vi "HoloPy_Example.vi"() -> ()   [LabVIEW 2023, in "holoPyTracks.lvlib"]
uses:
  holoPyTracks.lvlib
  subVis/HologramInfo.ctl
  subVis/analyse_parameters.ctl
panel:
  out "return value 2":sgl[][](array[numeric])
  out "2D Picture 3":picture
  out "2D Picture 2":picture
  out "return value":string
  out "data volume":cluster{"mean":dbl, "std var":dbl}
  out "2D Picture":picture
  in  "directory path":path=path "C:/TRAVAIL/developpement/imagesHolo/20um_bon_40X"
  in  "analyse parameters":T1={"propagation"={"distance ini"=0.0, "number of planes"=100, "step"=1e-06}, "Focus"={"Type"=enum."TENENGRAD", "Sum size"=20}, "Binarisation"={"Threshold ( N x Standard deviation)"=10.0, "Computed on"=enum."1st hologram"}, "CCL"={"Connectivity"=enum."6", "min voxel"=1.0, "max voxel"=1.0}, "Fourier BP filter (pix)"={"High pass (0=none)"=15.0, "Low Pass (0=none)"=125.0}} {"Fourier BP filter (pix)"."Low Pass (0=none)" format="%#_6e"; "CCL"."max voxel" min=1.0 max=100.0; "CCL"."min voxel" min=1.0 max=100.0; "Binarisation"."Threshold ( N x Standard deviation)" min=1.0 max=100.0; "Focus"."Sum size" min=1 max=100; "propagation"."step" format="%#_6e"; "propagation"."distance ini" format="%#_6e"}
  in  "Holo parameters":T2={"wavelength"=6.6e-07, "optical index"=1.33, "Holo size X"=1024, "Holo size Y"=1024, "pixel size"=7e-06, "objective magnification"=40.0} {"wavelength" format="%#_6e"}
  in  "image path":path=path "C:/TRAVAIL/developpement/imagesHolo/20um_bon_40X/20um_40x_int_.7ajp1c6t.000000.bmp"
  in  "error in (no error)":errorcluster
  in  "Python version":string="3.10"
  out "error out":errorcluster
  # "Python Node in holoPY.lvlib:HoloPy_Find_Features.vi->holoPY.lvlib:HoloPy_Example.vi<APPEND>\n\nModule Path: C:\\TRAVAIL\\developpement\\Holo_Python\\Holo_Python_Labview_wrapper.py\nFunction Name: LV_find_features\nPython returned the following error: <class 'ValueError'>\nOnly 6, 18, and 26 connectivities are supported for 3D images. Got: 0\n\n\nCall Stack information:\n  File \"C:\\TRAVAIL\\developpement\\Holo_Python\\Holo_Python_Labview_wrapper.py\", line 294, in LV_find_features\n    h_labels, number_of_labels, statsCCL3D = CCL3D(d_bin_volume_focus, d_volume_module, type_threshold.THRESHOLD, threshold, n_connectivity)\n  File \"C:\\TRAVAIL\\developpement\\Holo_Python\\CCL3D.py\", line 166, in CCL3D\n    labels, number_of_labels = cc3d.connected_components(h_bin_volum, connectivity=n_connectivity, out_dtype=np.uint16, return_N=True)\n  File \"cc3d.pyx\", line 273, in cc3d.connected_components\n\nValueError: Only 6, 18, and 26 connectivities are supported for 3D images. Got: 0"
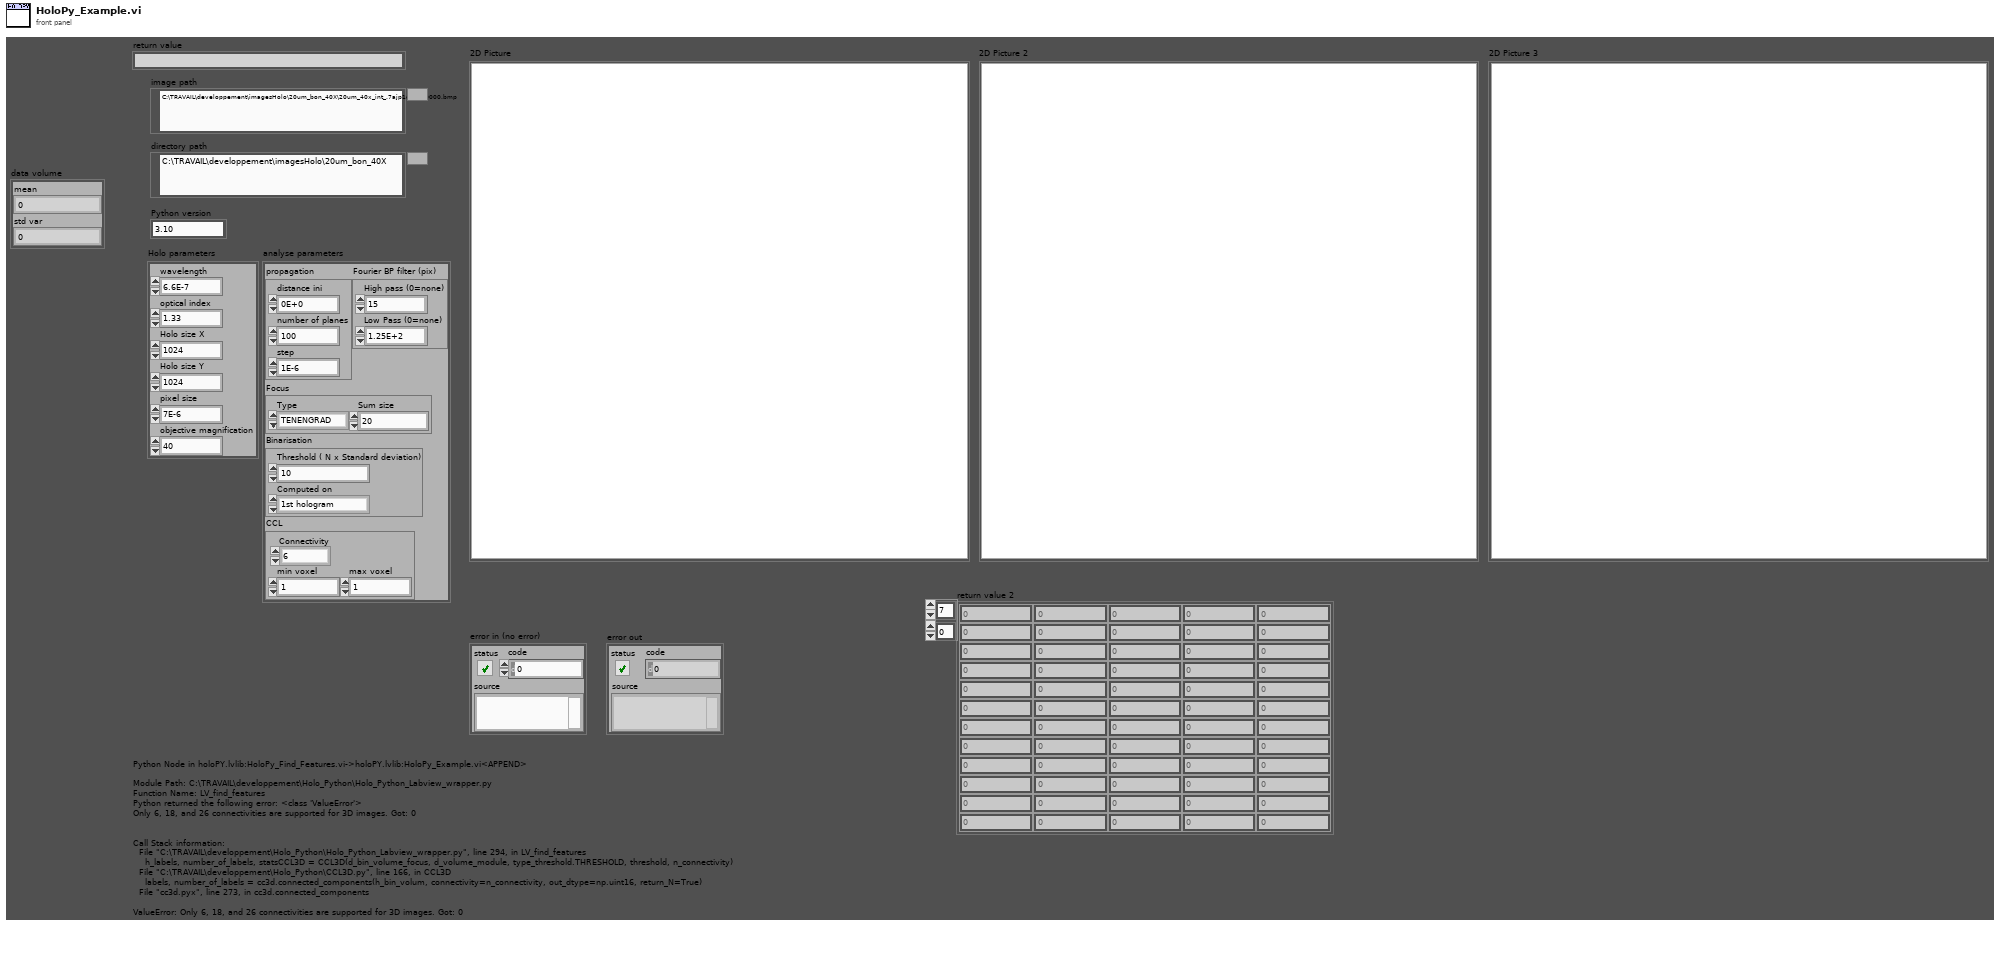
[diagram p1: front panel]
types:
  T1 = typedef "holoPyTracks.lvlib/analyse_parameters.ctl" = cluster{"propagation":cluster{"distance ini":dbl, "number of planes":i32, "step":dbl}, "Focus":cluster{"Type":enum16{"SUM_OF_INTENSITY", "SUM_OF_LAPLACIAN", "SUM_OF_VARIANCE", "TENENGRAD"}, "Sum size":i32}, "Binarisation":cluster{"Threshold ( N x Standard deviation)":dbl, "Computed on":enum16{"1st hologram", "each hologram"}}, "CCL":cluster{"Connectivity":enum16{"6", "18", "26"}, "min voxel":dbl, "max voxel":dbl}, "Fourier BP filter (pix)":cluster{"High pass (0=none)":dbl, "Low Pass (0=none)":dbl}}
  T2 = typedef "holoPyTracks.lvlib/HologramInfo.ctl" = cluster{"wavelength":sgl, "optical index":sgl, "Holo size X":i32, "Holo size Y":i32, "pixel size":sgl, "objective magnification":sgl}
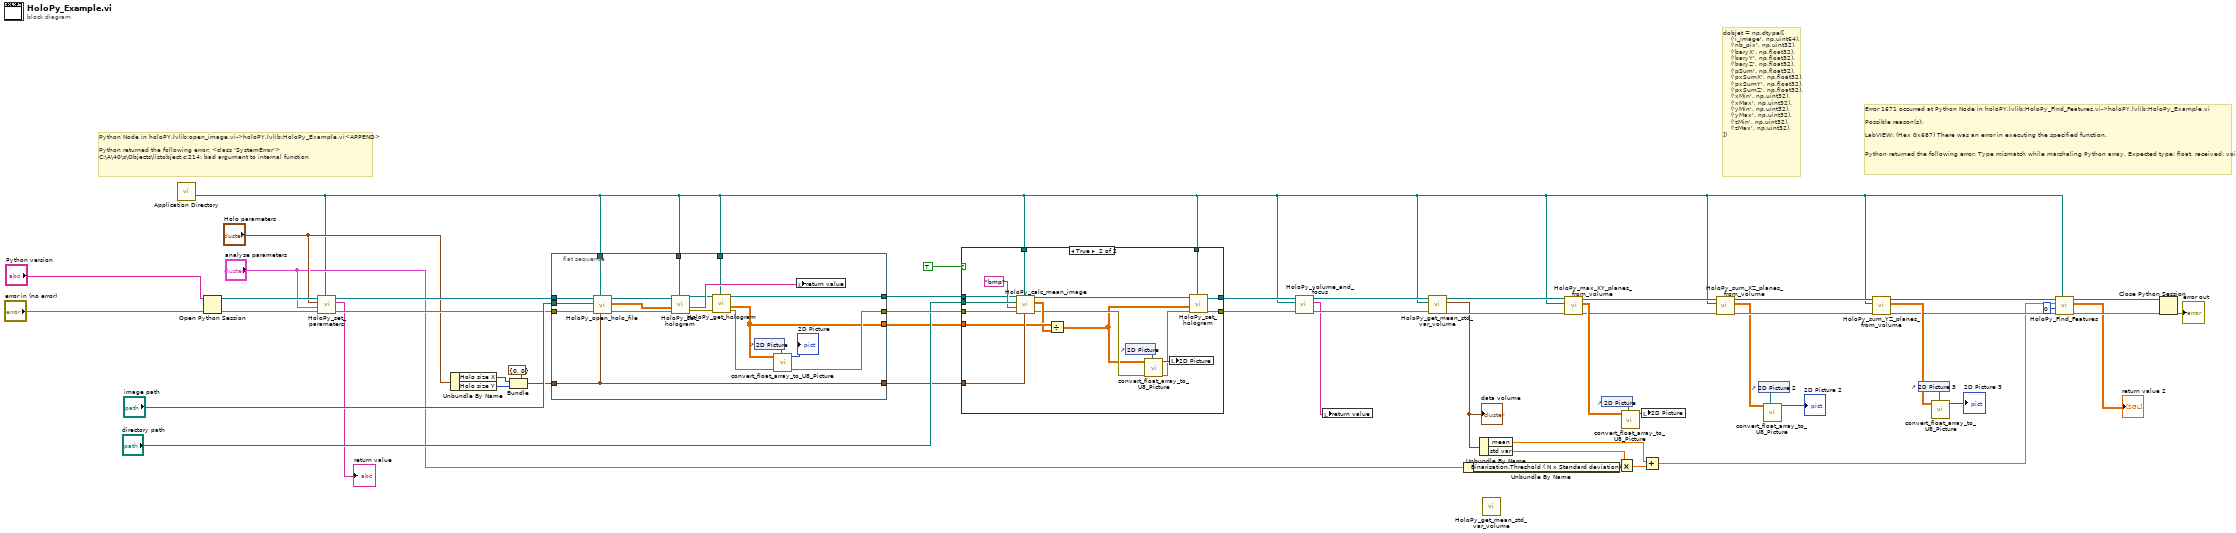
[diagram p0: block diagram]
diagram:
  # "Error 1671 occurred at Python Node in holoPY.lvlib:HoloPy_Find_Features.vi->holoPY.lvlib:HoloPy_Example.vi\n\nPossible reason(s):\n\nLabVIEW: (Hex 0x687) There was an error in executing the specified function.\n\n\nPython returned the following error: Type mismatch while marshaling Python array. Expected type: float, received: void."
  # "dobjet = np.dtype([\n    ('i_image', np.uint64),\n    ('nb_pix', np.uint32),\n    ('baryX', np.float32),\n    ('baryY', np.float32),\n    ('baryZ', np.float32),\n    ('pSum', np.float32),\n    ('pxSumX', np.float32),\n    ('pxSumY', np.float32),\n    ('pxSumZ', np.float32),\n    ('xMin', np.uint32),\n    ('xMax', np.uint32),\n    ('yMin', np.uint32),\n    ('yMax', np.uint32),\n    ('zMin', np.uint32),\n    ('zMax', np.uint32),\n])"
  # "Python Node in holoPY.lvlib:open_image.vi->holoPY.lvlib:HoloPy_Example.vi<APPEND>\n\nPython returned the following error: <class 'SystemError'>\nC:\\A\\40\\s\\Objects\\listobject.c:214: bad argument to internal function"
  n1 = call <vilib>:"Application Directory.vi"() -> ("Application Directory"=w6:path)
  n2 = Open Python Session(python version="Python version", 3:"error in (no error)") -> (session out=w43:refnum<k35>, error out=w42:errorcluster)  [unwired: 1 in]
  n3 = call "HoloPy_set_parameters.vi"(7:w6, "error in (no error)"=w42, "Parameters"="analyse parameters", 10:"Holo parameters", "session in"=w43) -> ("error out"=w41:errorcluster, "return value"=→"return value":string, "Refnum out"=w40:refnum<k35>)  [unwired: 4 in]
  n4 = Unbundle By Name("Holo parameters") -> ("Holo size X"=w21:i32, "Holo size Y"=w20:i32)
  n5 = Bundle(cluster=cluster{"image_size_X":i32, "image_size_Y":i32} {"image_size_X"=0, "image_size_Y"=0} ("imageSize"), "image_size_X"=w21, "image_size_Y"=w20) -> (w19:cluster{"image_size_X":i32, "image_size_Y":i32})
  n6 = flat-sequence {
    tunnel: [w61] -> w51
    tunnel: "image path" -> [w64]
    tunnel: w41 -> [w69]
    tunnel: w40 -> [w70]
    tunnel: w6 -> [w66]
    tunnel: w19 -> [w63]
    tunnel: w6 -> [w65]
    tunnel: [w63] -> w18
    tunnel: [w57] -> w17
    tunnel: w6 -> [w58]
    tunnel: [w55] -> w16
    frame #0 {
      n7 = call "HoloPy_open_holo_file.vi"("imageSize"=w63, 7:w66, "error in (no error)"=w69, "image path"=w64, "Refnum in"=w70) -> ("error out"=w67:errorcluster, "Array"=w62:sgl[][], "Refnum out"=w68:refnum<k35>)  [unwired: 4 in]
      n8 = call "HoloPy_set_hologram.vi"(7:w65, "error in (no error)"=w67, "HOLO_array"=w62, "Refnum in"=w68) -> ("error out"=w59:errorcluster, "return value"=w71:string, "Refnum out"=w60:refnum<k35>)  [unwired: 5 in]
      n9 = call "HoloPy_get_hologram.vi"(7:w58, "error in (no error)"=w59, "Refnum in"=w60) -> ("error out"=w56:errorcluster, "HOLO_array"=w57:sgl[][], "Refnum out"=w55:refnum<k35>)  [unwired: 6 in]
      n10 = control-ref of="2D Picture"() -> (w72:refnum<vi>)
      n11 = call "convert_float_array_to_U8_Picture.vi"("Pict Refnum"=w72, "error in (no error)"=w56, "HOLO"=w57) -> ("error out"=w61:errorcluster, "new picture"=→"2D Picture":picture)  [unwired: 7 in]
      n12 = local write "return value"(w71) -> ()
    }
  }
  n13 = case shown="True" TRUE {
    tunnel: w51 -> [w75 w92]
    tunnel: [w74 w84] -> w39
    tunnel: [w75 w85] -> w38
    tunnel: "directory path" -> [_ w88]
    tunnel: w6 -> [_ w89]
    tunnel: w18 -> [_ w86]
    tunnel: w6 -> [_ w83]
    tunnel: w17 -> [_ w81]
    tunnel: w16 -> [w74 w77]
    frame False {
    }
    frame True {
      n14 = call "HoloPy_calc_mean_image.vi"("imageSize"=w86, 7:w89, "error in (no error)"=w92, "imageFileExtension"="bmp", "directory path"=w88, "Refnum in"=w77) -> ("error out"=w79:errorcluster, "Array"=w80:sgl[][], "Refnum out"=w82:refnum<k35>)  [unwired: 3 in]
      n15 = Divide(x=w81, y=w80) -> (x/y=w76:sgl[][])
      n16 = control-ref of="2D Picture"() -> (w91:refnum<vi>)
      n17 = call "convert_float_array_to_U8_Picture.vi"("Pict Refnum"=w91, "error in (no error)"=w79, "HOLO"=w76) -> ("error out"=w78:errorcluster, "new picture"=w90:picture)  [unwired: 7 in]
      n18 = local write "2D Picture"(w90) -> ()
      n19 = call "HoloPy_set_hologram.vi"(7:w83, "error in (no error)"=w78, "HOLO_array"=w76, "Refnum in"=w82) -> ("error out"=w85:errorcluster, "Refnum out"=w84:refnum<k35>)  [unwired: 5 in, 1 out]
    }
  }
  n20 = call "HoloPy_volume_and_focus.vi"("error in (no error)"=w38, 10:w6, "Refnum in"=w39) -> ("error out"=w46:errorcluster, "return value"=w36:string, "Refnum out"=w47:refnum<k35>)  [unwired: 6 in]
  n21 = local write "return value"(w36) -> ()
  n22 = call "HoloPy_get_mean_std_var_volume.vi"("error in (no error)"=w46, 10:w6, "Refnum in"=w47) -> ("error out"=w44:errorcluster, "data volume"=w13:cluster{"mean":dbl, "std var":dbl}, "Refnum out"=w45:refnum<k35>)  [unwired: 6 in]
  "data volume" <- w13
  n23 = Unbundle By Name("analyse parameters") -> ("Binarisation.Threshold ( N x Standard deviation)"=w12:dbl)
  n24 = Unbundle By Name(w13) -> ("mean"=w9:dbl, "std var"=w11:dbl)
  n25 = call "HoloPy_get_mean_std_var_volume.vi"() -> ()  [unwired: 9 in, 3 out]
  n26 = call "HoloPy_max_XY_planes_from_volume.vi"("error in (no error)"=w44, 10:w6, "Refnum in"=w45) -> ("error out"=w32:errorcluster, "XY Plane"=w33:sgl[][], "Refnum out"=w31:refnum<k35>)  [unwired: 6 in]
  n27 = control-ref of="2D Picture"() -> (w34:refnum<vi>)
  n28 = Multiply(x=w11, y=w12) -> (x*y=w10:dbl)
  n29 = call "convert_float_array_to_U8_Picture.vi"("Pict Refnum"=w34, "HOLO"=w33) -> ("new picture"=w35:picture)  [unwired: 8 in, 1 out]
  n30 = local write "2D Picture"(w35) -> ()
  n31 = Add(x=w9, y=w10) -> (x+y=w3:dbl)
  n32 = call "HoloPy_sum_XZ_planes_from_volume.vi"("error in (no error)"=w32, 10:w6, "Refnum in"=w31) -> ("error out"=w29:errorcluster, "XZ Plane"=w26:sgl[][], "Refnum out"=w30:refnum<k35>)  [unwired: 6 in]
  n33 = control-ref of="2D Picture 2"() -> (w24:refnum<vi>)
  n34 = call "convert_float_array_to_U8_Picture.vi"("Pict Refnum"=w24, "HOLO"=w26) -> ("new picture"=→"2D Picture 2":picture)  [unwired: 8 in, 1 out]
  n35 = call "HoloPy_sum_YZ_planes_from_volume.vi"("error in (no error)"=w29, 10:w6, "Refnum in"=w30) -> ("error out"=w8:errorcluster, "YZ Plane"=w25:sgl[][], "Refnum out"=w7:refnum<k35>)  [unwired: 6 in]
  n36 = control-ref of="2D Picture 3"() -> (w23:refnum<vi>)
  n37 = call "convert_float_array_to_U8_Picture.vi"("Pict Refnum"=w23, "HOLO"=w25) -> ("new picture"=→"2D Picture 3":picture)  [unwired: 8 in, 1 out]
  n38 = call "HoloPy_Find_Features.vi"(7:w6, "error in (no error)"=w8, "imageNumber"=0, "Threshold"=w3, "Refnum in"=w7) -> ("error out"=w4:errorcluster, "FEATURES(µm)"=→"return value 2":sgl[][], "Refnum out"=w5:refnum<k35>)  [unwired: 4 in]
  n39 = Close Python Session(session in=w5, error in=w4) -> (11:→"error out":errorcluster)
